vi "BackUpMove.vi"() -> ()   [LabVIEW 2017]
uses:
  <vilib>/myRIO/Instrument Drivers/Onboard IO/DIO/typedefs/DIO Reference.ctl
  <vilib>/myRIO/Common/Instrument Driver Framework/Utilities/typedefs/myRIO Generic Hardware Reference.ctl
  <vilib>/myRIO/Common/Instrument Driver Framework/Utilities/typedefs/Hardware Version Enum.ctl
  <vilib>/myRIO/Common/Instrument Driver Framework/Utilities/typedefs/myRIO v1.0 Reference.ctl
  <vilib>/myRIO/Common/Instrument Driver Framework/Utilities/typedefs/Generic FPGA Reference.ctl
  <vilib>/myRIO/Common/Instrument Driver Framework/myRIO v1.0/DIO/typedefs/DIO Channels List.ctl
  <vilib>/myRIO/Common/Instrument Driver Framework/myRIO v1.0/DIO/typedefs/DIO Channels Enum.ctl
  <vilib>/userdefined/High Color/nirio_resource_hc.ctl
  <vilib>/userdefined/High Color/IMAQdx.ctl
  <vilib>/myRIO/Common/Instrument Driver Framework/Utilities/vis/Is FPGA Ref Available.vi
  <vilib>/myRIO/Common/Instrument Driver Framework/myRIO v1.0/DIO/vis/myRIO v1.1 Open DIO.vi
  <vilib>/myRIO/Instrument Drivers/Onboard IO/DIO/vis/Write.vi
  <vilib>/myRIO/Instrument Drivers/Onboard IO/DIO/vis/Read.vi
  <vilib>/myRIO/Common/Instrument Driver Framework/Utilities/vis/Validate Channels.vi
  <vilib>/myRIO/Common/Instrument Driver Framework/myRIO v1.0/DIO/vis/myRIO v1.0 Reserve DIO.vi
  <vilib>/myRIO/Common/Instrument Driver Framework/myRIO v1.0/Resource Manager/vis/myRIO v1.0 Reserve Channel List.vi
  <vilib>/myRIO/Common/Instrument Driver Framework/myRIO v1.0/DIO/vis/myRIO v1.0 Build MUX Configuration DIO.vi
  <vilib>/myRIO/Common/Instrument Driver Framework/myRIO v1.0/Resource Manager/vis/myRIO v1.0 Reserve Channel.vi
  <vilib>/myRIO/Common/Instrument Driver Framework/myRIO v1.0/Resource Manager/vis/myRIO v1.0 Unreserve Channel.vi
  <vilib>/myRIO/Common/Instrument Driver Framework/myRIO v1.0/Resource Manager/vis/myRIO v1.0 Create Configuration List.vi
  <vilib>/myRIO/Common/Instrument Driver Framework/myRIO v1.0/Resource Manager/vis/myRIO v1.0 Build Mutex Name.vi
  <vilib>/Utility/VariantDataType/GetNumericInfo.vi
  <vilib>/Utility/error.llb/Error Cluster From Error Code.vi
  <vilib>/myRIO/Common/Instrument Driver Framework/myRIO v1.0/myRIO v1.1 Open.vi
  <vilib>/myRIO/Common/Instrument Driver Framework/Utilities/vis/IO Manager.vi
  <vilib>/myRIO/Common/Instrument Driver Framework/Utilities/vis/Configuration Manager.vi
  <vilib>/myRIO/Common/Instrument Driver Framework/myRIO v1.0/Resource Manager/vis/myRIO v1.0 Configure IO.vi
  <vilib>/myRIO/Common/Instrument Driver Framework/myRIO v1.0/myRIO v1.0 Close.vi
  <vilib>/myRIO/Common/Instrument Driver Framework/myRIO v1.0/DIO/vis/myRIO v1.0 Write DIO.vi
  <vilib>/myRIO/Common/Instrument Driver Framework/myRIO v1.0/DIO/vis/myRIO v1.0 Read DIO.vi
  Global 5.vi
  <vilib>/myRIO/Express VI/Onboard Devices/LED/LED Express VI.xnode
  <vilib>/myRIO/Instrument Drivers/Onboard IO/DIO/vis/myRIO DIO Open.xnode
  <vilib>/myRIO/Express VI/Onboard Devices/Button/Button Express VI.xnode
  <vilib>/vision/NI_Vision_Development_Module.lvlib
  <vilib>/vision/driver/NI_Vision_Acquisition_Software.lvlib
  <vilib>/myRIO/Instrument Drivers/Onboard IO/DIO/DIO.lvlib
panel:
  out "x-y":dbl
  out "Count":T1(plugin-control)
  out "Extract":T1(plugin-control)
  out "Particle":T1(plugin-control)
  out "Threshold":T1(plugin-control)
  in  "Settings":T2={"Objects"=0, "Threshold"=128, "Reject Border"=FALSE, "Fill Holes"=FALSE, "Min Object Size"=FALSE, "Min Size"=3, "Max Object Size"=FALSE, "Max Size"=100, "Show Search Area"=FALSE, "Show Center"=TRUE, "Show Bounding Box"=TRUE} {"Objects" items=["Bright Objects", "Dark Objects"]; "Threshold" min=1 max=999999999 step=1; "Max Size" min=1 max=999999999 step=1; "Min Size" min=1 max=999999999 step=1}
  in  "Number of Objects":i32
  out "Number of Objects 2":i32
  out "ROI":T3
  out "Count Encode":dbl
  out "Status":string
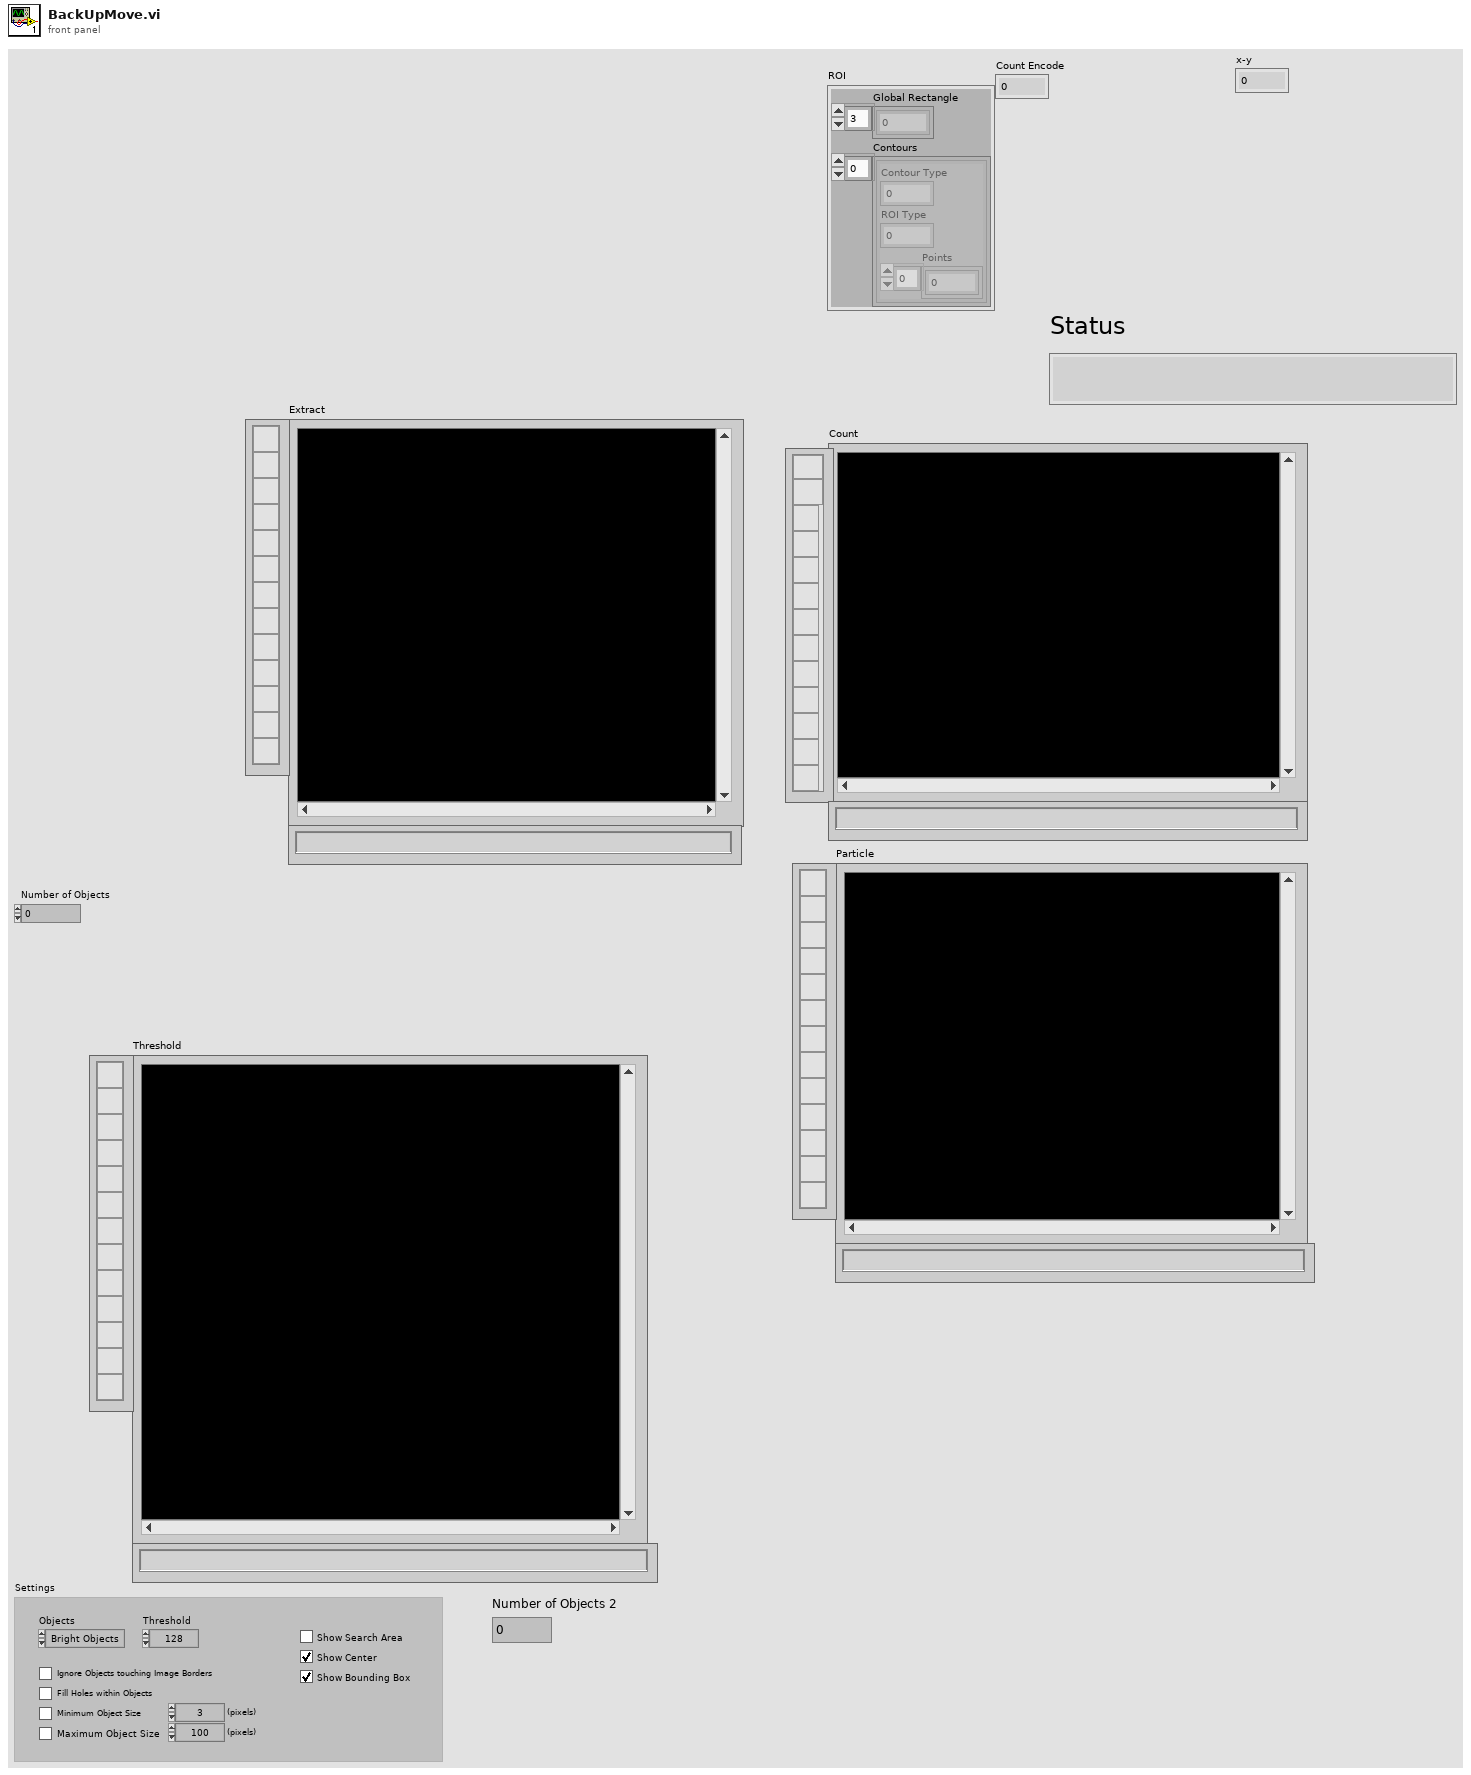
[diagram p1: front panel]
types:
  T1 = typedef "IMAQ Image.ctl" = refnum<image>
  T2 = cluster{"Objects":u16, "Threshold":i32, "Reject Border":bool, "Fill Holes":bool, "Min Object Size":bool, "Min Size":i32, "Max Object Size":bool, "Max Size":i32, "Show Search Area":bool, "Show Center":bool, "Show Bounding Box":bool}
  T3 = cluster{"Global Rectangle":i32[], "Contours":cluster{"Contour Type":u32, "ROI Type":u32, "Points":i32[]}[]}
  T4 = typedef "DIO.lvlib/DIO Reference.ctl" = cluster{"myRIO Reference":T5, "DIO Channels List":T9}
  T5 = typedef "myRIO Generic Hardware Reference.ctl" = cluster{"myRIO Model":T6, "myRIO Hardware Reference":T7}
  T6 = typedef "Hardware Version Enum.ctl" = enum16{"Unknown", "myRIO-1900", "myRIO-1950", "roboRIO", "NI ELVIS RIO CM"}
  T7 = typedef "myRIO v1.0 Reference.ctl" = cluster{"Generic FPGA Reference":T8, "Allow multiple opens":bool}
  T8 = typedef "Generic FPGA Reference.ctl" = refnum<k20>
  T9 = typedef "DIO Channels List.ctl" = T10[]
  T10 = typedef "DIO Channels Enum.ctl" = enum16{"Not Connected", "C/DIO0", "C/DIO1", "C/DIO2", "C/DIO3", "C/DIO4", "C/DIO5", "C/DIO6", "C/DIO7", "A/DIO0", "A/DIO1", "A/DIO2", "A/DIO3", "A/DIO4", "A/DIO5", "A/DIO6", "A/DIO7", "A/DIO8", "A/DIO9", "A/DIO10", "A/DIO11", "A/DIO12", "A/DIO13", "A/DIO14", "A/DIO15", "B/DIO0", "B/DIO1", "B/DIO2", "B/DIO3", "B/DIO4", "B/DIO5", "B/DIO6", "B/DIO7", "B/DIO8", "B/DIO9", "B/DIO10", "B/DIO11", "B/DIO12", "B/DIO13", "B/DIO14", "B/DIO15", "LED0", "LED1", "LED2", "LED3", "Button0", "DIO/DIO0", "DIO/DIO1", "DIO/DIO2", "DIO/DIO3", "DIO/DIO4", "DIO/DIO5", "DIO/DIO6", "DIO/DIO7", "DIO/DIO8", "DIO/DIO9", "SPI/CS0", "SPI/CS1", "SPI/CS2", "SPI/CS3", "LED RADIO (Green)", "LED RADIO (Red)", "LED COMM (Green)", "LED COMM (Red)", "LED MODE (Green)", "LED MODE (Red)"}
  T11 = typedef "nirio_resource_hc.ctl" = tag
  T12 = typedef "IMAQdx.ctl" = refnum<k21>
diagram:
  n1 = flat-sequence {
    tunnel: [w75] -> w1
    tunnel: [w156] -> w74
    tunnel: [w155] -> w73
    tunnel: [w152] -> w72
    tunnel: w1 -> [w150]
    tunnel: [w202] -> w71
    tunnel: [w201] -> w70
    tunnel: w74 -> [w202]
    tunnel: w73 -> [w201]
    tunnel: w72 -> [w200]
    tunnel: [w199] -> w69
    tunnel: w71 -> [w211]
    tunnel: w70 -> [w210]
    tunnel: [w211] -> w68
    tunnel: [w210] -> w67
    tunnel: w69 -> [w209]
    tunnel: [w208] -> w66
    tunnel: [w221] -> w65
    tunnel: [w220] -> w64
    tunnel: w68 -> [w221]
    tunnel: w67 -> [w220]
    tunnel: w66 -> [w217]
    tunnel: [w215] -> w63
    tunnel: w65 -> [w230]
    tunnel: w64 -> [w229]
    tunnel: [w230] -> w61
    tunnel: [w229] -> w62
    tunnel: w63 -> [w228]
    tunnel: [w227] -> w60
    tunnel: w62 -> [w237]
    tunnel: [w237] -> w59
    tunnel: w61 -> [w236]
    tunnel: [w236] -> w58
    tunnel: [w234] -> w57
    tunnel: w60 -> [w234]
    tunnel: w59 -> [w244]
    tunnel: w58 -> [w243]
    tunnel: [w244] -> w56
    tunnel: [w243] -> w55
    tunnel: w57 -> [w240]
    tunnel: [w238] -> w54
    tunnel: w56 -> [w252]
    tunnel: w55 -> [w253]
    tunnel: [w253] -> w53
    tunnel: [w252] -> w52
    tunnel: w54 -> [w251]
    tunnel: [w250] -> w51
    tunnel: [w260] -> w50
    tunnel: w53 -> [w260]
    tunnel: [w259] -> w49
    tunnel: w52 -> [w259]
    tunnel: [w257] -> w48
    tunnel: w51 -> [w257]
    tunnel: [w264] -> w47
    tunnel: [w266] -> w46
    tunnel: w50 -> [w266]
    tunnel: w49 -> [w264]
    tunnel: w48 -> [w263]
    tunnel: [w262] -> w45
    tunnel: w47 -> [w311]
    tunnel: w46 -> [w312]
    tunnel: [w312] -> w44
    tunnel: [w311] -> w43
    tunnel: w45 -> [w310]
    tunnel: [w309] -> w42
    tunnel: [w355] -> w41
    tunnel: [w356] -> w40
    tunnel: w44 -> [w356]
    tunnel: w43 -> [w355]
    tunnel: w42 -> [w353]
    tunnel: [w351] -> w39
    tunnel: w41 -> [w364]
    tunnel: w40 -> [w365]
    tunnel: w39 -> [w367]
    tunnel: [w366] -> w38
    tunnel: [w365] -> w37
    tunnel: [w364] -> w36
    tunnel: [w372] -> w35
    tunnel: [w373] -> w34
    tunnel: w38 -> [w376]
    tunnel: w37 -> [w375]
    tunnel: w36 -> [w374]
    tunnel: [w371] -> w33
    tunnel: [w435] -> w32
    tunnel: [w436] -> w31
    tunnel: w35 -> [w435]
    tunnel: w34 -> [w433]
    tunnel: [w431] -> w30
    tunnel: w33 -> [w436]
    tunnel: w32 -> [w446]
    tunnel: w31 -> [w445]
    tunnel: [w445] -> w29
    tunnel: [w446] -> w28
    tunnel: [w445] -> w27
    tunnel: w30 -> [w444]
    tunnel: [w443] -> w26
    tunnel: w29 -> [_]
    tunnel: w28 -> [w452]
    tunnel: [w452] -> w25
    tunnel: [w451] -> w24
    tunnel: w27 -> [w451]
    tunnel: w26 -> [w450]
    tunnel: [w450] -> w23
    tunnel: w25 -> [w458]
    tunnel: w24 -> [w459]
    tunnel: [w459] -> w22
    tunnel: [w458] -> w21
    tunnel: w23 -> [w456]
    tunnel: [w454] -> w20
    tunnel: w22 -> [w467]
    tunnel: w21 -> [w466]
    tunnel: w20 -> [w469]
    tunnel: [w468] -> w4
    tunnel: [w467] -> w3
    tunnel: [w466] -> w2
    tunnel: [w478] -> w19
    tunnel: [w473] -> w18
    tunnel: [w474] -> w17
    tunnel: w4 -> [w475]
    tunnel: w3 -> [w474]
    tunnel: w2 -> [w473]
    tunnel: w19 -> [w490]
    tunnel: [w489] -> w16
    tunnel: w18 -> [w488]
    tunnel: [w488] -> w15
    tunnel: w17 -> [w487]
    tunnel: [w487] -> w14
    tunnel: w16 -> [w495]
    tunnel: w15 -> [w497]
    tunnel: w14 -> [w496]
    tunnel: [w497] -> w13
    tunnel: [w496] -> w12
    tunnel: [w495] -> w11
    tunnel: w13 -> [w508]
    tunnel: [w508] -> w10
    tunnel: w12 -> [w507]
    tunnel: [w507] -> w9
    tunnel: w11 -> [w506]
    tunnel: [w505] -> w8
    tunnel: w10 -> [w515]
    tunnel: w9 -> [w514]
    tunnel: w8 -> [w517]
    tunnel: [w515] -> w7
    tunnel: [w514] -> w6
    tunnel: [w513] -> w5
    tunnel: w7 -> [w563]
    tunnel: w6 -> [w562]
    tunnel: w5 -> [w561]
    frame #0 {
      n2 = while {
        tunnel: [w76] -> w75
        stop <- w78 stop-if-true
        n3 = xnode "Start"("LED0"=TRUE) -> ("error out"=w77:errorcluster)  [unwired: 1 in]
        n4 = xnode "Button"("error in (no error)"=w77) -> ("Value"=w78:bool, "error out"=w76:errorcluster)
      }
    }
    frame #1 {
      w156 = tag "B/I2C" ("myRIO MXP Port A/B")
      w155 = u8 1 ("Controller ID#  (I2C Address)")
      # "enable"
      n5 = Wait (ms)(milliseconds to wait=u32 1000) -> ()  [unwired: 1 out]
      n6 = local write "Status"("Starting" ("Status")) -> ()
      n7 = xnode "Start 2"("LED0"=FALSE) -> ()  [unwired: 1 in, 1 out]
      n8 = call <vilib>:"TETRIX_Enable_DC_Controller_myRIO.vi"("myRIO MXP Port A/B"=w156, "Controller ID#  (I2C Address)"=w155, "Error/Flow In"=w150) -> ("Error/Flow Out"=w154:errorcluster)  [unwired: 4 in]
      n9 = call <vilib>:"TETRIX_Motor_Invert_myRIO.vi"("myRIO MXP Port A/B"=w156, "Invert State"=TRUE, "Select Channel"="Motor 1", "Controller ID#  (I2C Address)"=w155) -> ()  [unwired: 3 in, 1 out]
      n10 = call <vilib>:"TETRIX_Reset_Encoders_myRIO.vi"("myRIO MXP Port A/B"=w156, "Select Encoder"="Encoders 1 and 2", "Controller ID#  (I2C Address)"=w155, "Error/Flow In"=w154) -> ("Error/Flow Out"=w153:errorcluster)  [unwired: 3 in]
      n11 = call <vilib>:"TETRIX_Stop_Motors_myRIO.vi"("myRIO MXP Port A/B"=w156, "Stop Mode"="Brake", "Select Channel"="Both Motors", "Controller ID#  (I2C Address)"=w155, "Error/Flow In"=w153) -> ("Error/Flow Out"=w152:errorcluster)  [unwired: 2 in]
    }
    frame #2 {
      w204 = 700 ("Motor 2 Encoder Target")
      w206 = i16 200 ("Motor 1 Contant Speed (Degrees per Second)")
      # "fate 1 start position"
      n12 = Wait (ms)(milliseconds to wait=u32 5500) -> ()  [unwired: 1 out]
      n13 = call <vilib>:"TETRIX_Set_Motor_Target(s)_myRIO.vi"("Motor 2 Encoder Target"=w204, "Motor 1 Encoder Target"=w204, "myRIO MXP Port A/B"=w202, "Controller ID#  (I2C Address)"=w201, "Motor 2 Constant Speed (Degrees per Second)"=w206, "Motor 1 Contant Speed (Degrees per Second)"=w206, "Encoder Units"="Degrees", "Error/Flow In"=w200) -> ("Error/Flow Out"=w199:errorcluster)  [unwired: 1 in]
      "Status" <- "Phase 1" ("Status")
    }
    frame #3 {
      n14 = Wait (ms)(milliseconds to wait=u32 500) -> ()  [unwired: 1 out]
      n15 = call <vilib>:"TETRIX_Stop_Motors_myRIO.vi"("myRIO MXP Port A/B"=w211, "Stop Mode"="Brake", "Select Channel"="Both Motors", "Controller ID#  (I2C Address)"=w210, "Error/Flow In"=w209) -> ("Error/Flow Out"=w208:errorcluster)  [unwired: 2 in]
    }
    frame #4 {
      w226 = i16 100 ("Motor 1 Contant Speed (Degrees per Second)")
      # "fate 2 catch ball"
      n16 = Wait (ms)(milliseconds to wait=u32 3000) -> ()  [unwired: 1 out]
      n17 = local write "Status"("Turning" ("Status")) -> ()
      n18 = call <vilib>:"TETRIX_Reset_Encoders_myRIO.vi"("myRIO MXP Port A/B"=w221, "Select Encoder"="Encoders 1 and 2", "Controller ID#  (I2C Address)"=w220, "Error/Flow In"=w217) -> ("Error/Flow Out"=w216:errorcluster)  [unwired: 3 in]
      n19 = call <vilib>:"TETRIX_Set_Motor_Target(s)_myRIO.vi"("Motor 2 Encoder Target"=300 ("Motor 1 Encoder Target"), "Motor 1 Encoder Target"=-290, "myRIO MXP Port A/B"=w221, "Controller ID#  (I2C Address)"=w220, "Motor 2 Constant Speed (Degrees per Second)"=w226, "Motor 1 Contant Speed (Degrees per Second)"=w226, "Encoder Units"="Degrees", "Error/Flow In"=w216) -> ("Error/Flow Out"=w215:errorcluster)  [unwired: 1 in]
    }
    frame #5 {
      n20 = Wait (ms)(milliseconds to wait=u32 500) -> ()  [unwired: 1 out]
      n21 = call <vilib>:"TETRIX_Stop_Motors_myRIO.vi"("myRIO MXP Port A/B"=w230, "Stop Mode"="Brake", "Select Channel"="Both Motors", "Controller ID#  (I2C Address)"=w229, "Error/Flow In"=w228) -> ("Error/Flow Out"=w227:errorcluster)  [unwired: 2 in]
    }
    frame #6 {
      n22 = local write "Status"("Move Gripper" ("Status")) -> ()
      n23 = call "ServoPickup.vi"() -> ()  [unwired: 12 in]
    }
    frame #7 {
      w246 = i16 100 ("Motor 1 Contant Speed (Degrees per Second)")
      n24 = Wait (ms)(milliseconds to wait=u32 5000) -> ()  [unwired: 1 out]
      n25 = local write "Status"("Moving to catch" ("Status")) -> ()
      n26 = call <vilib>:"TETRIX_Reset_Encoders_myRIO.vi"("myRIO MXP Port A/B"=w243, "Select Encoder"="Encoders 1 and 2", "Controller ID#  (I2C Address)"=w244, "Error/Flow In"=w240) -> ("Error/Flow Out"=w239:errorcluster)  [unwired: 3 in]
      n27 = call <vilib>:"TETRIX_Set_Motor_Target(s)_myRIO.vi"("Motor 2 Encoder Target"=420 ("Motor 1 Encoder Target"), "Motor 1 Encoder Target"=420, "myRIO MXP Port A/B"=w243, "Controller ID#  (I2C Address)"=w244, "Motor 2 Constant Speed (Degrees per Second)"=w246, "Motor 1 Contant Speed (Degrees per Second)"=w246, "Encoder Units"="Degrees", "Error/Flow In"=w239) -> ("Error/Flow Out"=w238:errorcluster)  [unwired: 1 in]
    }
    frame #8 {
      n28 = Wait (ms)(milliseconds to wait=u32 500) -> ()  [unwired: 1 out]
      n29 = call <vilib>:"TETRIX_Stop_Motors_myRIO.vi"("myRIO MXP Port A/B"=w253, "Stop Mode"="Brake", "Select Channel"="Both Motors", "Controller ID#  (I2C Address)"=w252, "Error/Flow In"=w251) -> ("Error/Flow Out"=w250:errorcluster)  [unwired: 2 in]
    }
    frame #9 {
      n30 = local write "Status"("Catching" ("Status")) -> ()
      n31 = call "PickBall.vi"() -> ()  [unwired: 12 in]
    }
    frame #10 {
      w269 = i16 100 ("Motor 1 Contant Speed (Degrees per Second)")
      n32 = Wait (ms)(milliseconds to wait=u32 4200) -> ()  [unwired: 1 out]
      n33 = xnode "LED"("LED1"=TRUE) -> ()  [unwired: 1 in, 1 out]
      n34 = call <vilib>:"TETRIX_Set_Motor_Target(s)_myRIO.vi"("Motor 2 Encoder Target"=300 ("Motor 1 Encoder Target"), "Motor 1 Encoder Target"=300, "myRIO MXP Port A/B"=w266, "Controller ID#  (I2C Address)"=w264, "Motor 2 Constant Speed (Degrees per Second)"=w269, "Motor 1 Contant Speed (Degrees per Second)"=w269, "Encoder Units"="Degrees", "Error/Flow In"=w263) -> ("Error/Flow Out"=w262:errorcluster)  [unwired: 1 in]
      n35 = local write "Status"("Moving to Bowling" ("Status")) -> ()
      n36 = call <vilib>:"TETRIX_Reset_Encoders_myRIO.vi"("myRIO MXP Port A/B"=w266, "Select Encoder"="Encoders 1 and 2", "Controller ID#  (I2C Address)"=w264) -> ()  [unwired: 4 in, 1 out]
    }
    frame #11 {
      # "end fate2"
      n37 = Wait (ms)(milliseconds to wait=u32 500) -> ()  [unwired: 1 out]
      n38 = xnode "LED 2"("LED1"=FALSE) -> ()  [unwired: 1 in, 1 out]
      n39 = call <vilib>:"TETRIX_Stop_Motors_myRIO.vi"("myRIO MXP Port A/B"=w312, "Stop Mode"="Brake", "Select Channel"="Both Motors", "Controller ID#  (I2C Address)"=w311, "Error/Flow In"=w310) -> ("Error/Flow Out"=w309:errorcluster)  [unwired: 2 in]
    }
    frame #12 {
      w360 = i16 100 ("Motor 2 Constant Speed (Degrees per Second)")
      # "fate 3  go to shoot ball position"
      n40 = Wait (ms)(milliseconds to wait=u32 3000) -> ()  [unwired: 1 out]
      n41 = local write "Status"("Phase 3 Turning" ("Status")) -> ()
      n42 = call <vilib>:"TETRIX_Reset_Encoders_myRIO.vi"("myRIO MXP Port A/B"=w356, "Select Encoder"="Encoders 1 and 2", "Controller ID#  (I2C Address)"=w355, "Error/Flow In"=w353) -> ("Error/Flow Out"=w352:errorcluster)  [unwired: 3 in]
      n43 = call <vilib>:"TETRIX_Set_Motor_Target(s)_myRIO.vi"("Motor 2 Encoder Target"=300, "Motor 1 Encoder Target"=-315, "myRIO MXP Port A/B"=w356, "Controller ID#  (I2C Address)"=w355, "Motor 2 Constant Speed (Degrees per Second)"=w360, "Motor 1 Contant Speed (Degrees per Second)"=w360, "Encoder Units"="Degrees", "Error/Flow In"=w352) -> ("Error/Flow Out"=w351:errorcluster)  [unwired: 1 in]
    }
    frame #13 {
      n44 = Wait (ms)(milliseconds to wait=u32 500) -> ()  [unwired: 1 out]
      n45 = global write "Global 5.vi" "Count Encode"(50.0 ("Count Encode")) -> ()
      n46 = call <vilib>:"TETRIX_Stop_Motors_myRIO.vi"("myRIO MXP Port A/B"=w365, "Stop Mode"="Brake", "Select Channel"="Both Motors", "Controller ID#  (I2C Address)"=w364, "Error/Flow In"=w367) -> ("Error/Flow Out"=w366:errorcluster)  [unwired: 2 in]
    }
    frame #14 {
      (unwired) "im0" ("Image Name")
      n47 = call "IMAQ Create"("Image Name"="im0") -> ("New Image"=w380:T1)  [unwired: 4 in, 1 out]
      n48 = call "IMAQ Create"("Image Name"="im1") -> ("New Image"=w378:T1)  [unwired: 4 in, 1 out]
      n49 = while {
        tunnel: w380 -> [w408]
        tunnel: w378 -> [w405]
        tunnel: w374 -> [w401]
        tunnel: w376 -> [w389]
        tunnel: w375 -> [w384]
        tunnel: [w387] -> w373
        tunnel: [w385] -> w372
        tunnel: [w382] -> w371
        stop <- w399 stop-if-true
        w409 = u16 1 items=["RGB", "HSL", "HSV", "HSI"] ("Color Mode")
        n50 = flat-sequence {
          tunnel: w401 -> [w413]
          tunnel: w389 -> [w418]
          tunnel: [w416] -> w388
          tunnel: [w413] -> w386
          tunnel: w384 -> [w412]
          tunnel: [w412] -> w383
          tunnel: w388 -> [w427]
          tunnel: [w426] -> w387
          tunnel: w386 -> [w425]
          tunnel: [w425] -> w385
          tunnel: w383 -> [w424]
          tunnel: [w424] -> w382
          frame #0 {
            w415 = 50 ("Motor 1 Encoder Target")
            w421 = i16 100 ("Motor 1 Contant Speed (Degrees per Second)")
            n51 = global read "Global 5.vi" "Count Encode"() -> (w419:dbl)
            n52 = Wait (ms)(milliseconds to wait=u32 500 ("millisecond timer value")) -> ()  [unwired: 1 out]
            n53 = Add(x=50.0, y=w419) -> (x+y=w411:dbl)
            "Count Encode" <- w411
            n54 = call <vilib>:"TETRIX_Reset_Encoders_myRIO.vi"("myRIO MXP Port A/B"=w412, "Select Encoder"="Encoders 1 and 2", "Controller ID#  (I2C Address)"=w413, "Error/Flow In"=w418) -> ("Error/Flow Out"=w417:errorcluster)  [unwired: 3 in]
            n55 = call <vilib>:"TETRIX_Set_Motor_Target(s)_myRIO.vi"("Motor 2 Encoder Target"=w415, "Motor 1 Encoder Target"=w415, "myRIO MXP Port A/B"=w412, "Controller ID#  (I2C Address)"=w413, "Motor 2 Constant Speed (Degrees per Second)"=w421, "Motor 1 Contant Speed (Degrees per Second)"=w421, "Encoder Units"="Degrees", "Error/Flow In"=w417) -> ("Error/Flow Out"=w416:errorcluster)  [unwired: 1 in]
            n56 = global write "Global 5.vi" "Count Encode"(w411) -> ()
          }
          frame #1 {
            n57 = Wait (ms)(milliseconds to wait=u32 500 ("millisecond timer value")) -> ()  [unwired: 1 out]
            n58 = call <vilib>:"TETRIX_Stop_Motors_myRIO.vi"("myRIO MXP Port A/B"=w424, "Stop Mode"="Brake", "Select Channel"="Both Motors", "Controller ID#  (I2C Address)"=w425, "Error/Flow In"=w427) -> ("Error/Flow Out"=w426:errorcluster)  [unwired: 2 in]
          }
        }
        n59 = property on="Count" class="ImageControl"() -> ("ROI"=→"ROI":T3)  [unwired: 2 in, 2 out]
        n60 = call <vilib>:"IMAQdx Snap2.vi"("Image In"=w408, "Session In"=T12 "cam0") -> ("Image Out"=w410:T1)  [unwired: 7 in, 2 out]
        n61 = call "IMAQ ExtractColorPlanes"("Blue or Luma or Val or Inten Plane"=w405, "Color Mode"=w409, "Image Src"=w410) -> ("Blue or Luma or Val or Inten Plane out"=w406:T1)  [unwired: 5 in, 3 out]
        n62 = call "IMAQ Rotate"("Angle (degrees)"=sgl -2.3, "Image Src"=w406) -> ("Image Dst Out"=w395:T1)  [unwired: 8 in, 1 out]
        "Count" <- w395
        n63 = call "IMAQ Extract 2"("Optional Rectangle"=i32[] [327, 228, 351, 263], "Image Src"=w395) -> ("Image Dst Out"=w404:T1)  [unwired: 8 in, 1 out]
        "Extract" <- w404
        "Particle" <- w404
        n64 = global read "Global 5.vi" "Count Encode"() -> (w398:dbl)
        n65 = call "IMAQ Count Objects 2"("Settings"="Settings", "Image"=w404) -> ("Number of Objects"=w392:i32, "Image Out"=→"Threshold":T1)  [unwired: 5 in, 3 out]
        "Number of Objects 2" <- w392
        n66 = Greater?(x=w392, y=2) -> (0:w393:bool)
        n67 = Greater Or Equal?(x=w398, y=1200.0) -> (x >= y?=w396:bool)
        n68 = Or(x=w393, y=w396) -> (x .or. y?=w399:bool)
      }
      n69 = local write "Status"("IMAQ Start" ("Status")) -> ()
    }
    frame #15 {
      w441 = i16 100 ("Motor 1 Contant Speed (Degrees per Second)")
      n70 = Wait (ms)(milliseconds to wait=u32 3000) -> ()  [unwired: 1 out]
      n71 = local write "Status"("Turning to shoot" ("Status")) -> ()
      n72 = call <vilib>:"TETRIX_Reset_Encoders_myRIO.vi"("myRIO MXP Port A/B"=w436, "Select Encoder"="Encoders 1 and 2", "Controller ID#  (I2C Address)"=w435, "Error/Flow In"=w433) -> ("Error/Flow Out"=w432:errorcluster)  [unwired: 3 in]
      n73 = call <vilib>:"TETRIX_Set_Motor_Target(s)_myRIO.vi"("Motor 2 Encoder Target"=-285, "Motor 1 Encoder Target"=290, "myRIO MXP Port A/B"=w436, "Controller ID#  (I2C Address)"=w435, "Motor 2 Constant Speed (Degrees per Second)"=w441, "Motor 1 Contant Speed (Degrees per Second)"=w441, "Encoder Units"="Degrees", "Error/Flow In"=w432) -> ("Error/Flow Out"=w431:errorcluster)  [unwired: 1 in]
    }
    frame #16 {
      n74 = Wait (ms)(milliseconds to wait=u32 500) -> ()  [unwired: 1 out]
      n75 = call <vilib>:"TETRIX_Stop_Motors_myRIO.vi"("myRIO MXP Port A/B"=w445, "Stop Mode"="Brake", "Select Channel"="Both Motors", "Controller ID#  (I2C Address)"=w446, "Error/Flow In"=w444) -> ("Error/Flow Out"=w443:errorcluster)  [unwired: 2 in]
    }
    frame #17 {
      # "fate 4 shoot ball"
      n76 = local write "Status"(" Shooting" ("Status")) -> ()
      n77 = call "Shoot.vi"() -> ()  [unwired: 12 in]
    }
    frame #18 {
      w464 = i16 100 ("Motor 1 Contant Speed (Degrees per Second)")
      n78 = Wait (ms)(milliseconds to wait=u32 3000) -> ()  [unwired: 1 out]
      n79 = local write "Status"("Turning to Check" ("Status")) -> ()
      n80 = call <vilib>:"TETRIX_Reset_Encoders_myRIO.vi"("myRIO MXP Port A/B"=w459, "Select Encoder"="Encoders 1 and 2", "Controller ID#  (I2C Address)"=w458, "Error/Flow In"=w456) -> ("Error/Flow Out"=w455:errorcluster)  [unwired: 3 in]
      n81 = call <vilib>:"TETRIX_Set_Motor_Target(s)_myRIO.vi"("Motor 2 Encoder Target"=300, "Motor 1 Encoder Target"=-285, "myRIO MXP Port A/B"=w459, "Controller ID#  (I2C Address)"=w458, "Motor 2 Constant Speed (Degrees per Second)"=w464, "Motor 1 Contant Speed (Degrees per Second)"=w464, "Encoder Units"="Degrees", "Error/Flow In"=w455) -> ("Error/Flow Out"=w454:errorcluster)  [unwired: 1 in]
    }
    frame #19 {
      n82 = Wait (ms)(milliseconds to wait=u32 500) -> ()  [unwired: 1 out]
      n83 = call <vilib>:"TETRIX_Stop_Motors_myRIO.vi"("myRIO MXP Port A/B"=w467, "Stop Mode"="Brake", "Select Channel"="Both Motors", "Controller ID#  (I2C Address)"=w466, "Error/Flow In"=w469) -> ("Error/Flow Out"=w468:errorcluster)  [unwired: 2 in]
    }
    frame #20 {
      w484 = i16 200 ("Motor 1 Contant Speed (Degrees per Second)")
      n84 = call <vilib>:"TETRIX_Reset_Encoders_myRIO.vi"("myRIO MXP Port A/B"=w474, "Select Encoder"="Encoders 1 and 2", "Controller ID#  (I2C Address)"=w473, "Error/Flow In"=w475) -> ("Error/Flow Out"=w485:errorcluster)  [unwired: 3 in]
      n85 = Wait (ms)(milliseconds to wait=u32 5000) -> ()  [unwired: 1 out]
      n86 = global read "Global 5.vi" "Count Encode"() -> (w481:dbl)
      n87 = local write "Status"("Encode to Home " ("Status")) -> ()
      n88 = Subtract(x=870.0, y=w481) -> (x-y=w479:dbl)
      "x-y" <- w479
      n89 = call <vilib>:"TETRIX_Set_Motor_Target(s)_myRIO.vi"("Motor 2 Encoder Target"=w479, "Motor 1 Encoder Target"=w479, "myRIO MXP Port A/B"=w474, "Controller ID#  (I2C Address)"=w473, "Motor 2 Constant Speed (Degrees per Second)"=w484, "Motor 1 Contant Speed (Degrees per Second)"=w484, "Encoder Units"="Degrees", "Error/Flow In"=w485) -> ("Error/Flow Out"=w478:errorcluster)  [unwired: 1 in]
    }
    frame #21 {
      n90 = call <vilib>:"TETRIX_Stop_Motors_myRIO.vi"("myRIO MXP Port A/B"=w487, "Stop Mode"="Brake", "Select Channel"="Both Motors", "Controller ID#  (I2C Address)"=w488, "Error/Flow In"=w490) -> ("Error/Flow Out"=w489:errorcluster)  [unwired: 2 in]
      n91 = Wait (ms)(milliseconds to wait=u32 500) -> ()  [unwired: 1 out]
    }
    frame #22 {
      w502 = i16 100 ("Motor 1 Contant Speed (Degrees per Second)")
      n92 = call <vilib>:"TETRIX_Reset_Encoders_myRIO.vi"("myRIO MXP Port A/B"=w496, "Select Encoder"="Encoders 1 and 2", "Controller ID#  (I2C Address)"=w497, "Error/Flow In"=w495) -> ("Error/Flow Out"=w499:errorcluster)  [unwired: 3 in]
      n93 = local write "Status"("Turning" ("Status")) -> ()
      n94 = Wait (ms)(milliseconds to wait=u32 4500) -> ()  [unwired: 1 out]
      n95 = call <vilib>:"TETRIX_Set_Motor_Target(s)_myRIO.vi"("Motor 2 Encoder Target"=290, "Motor 1 Encoder Target"=-295, "myRIO MXP Port A/B"=w496, "Controller ID#  (I2C Address)"=w497, "Motor 2 Constant Speed (Degrees per Second)"=w502, "Motor 1 Contant Speed (Degrees per Second)"=w502, "Encoder Units"="Degrees", "Error/Flow In"=w499) -> ()  [unwired: 1 in, 1 out]
    }
    frame #23 {
      n96 = call <vilib>:"TETRIX_Stop_Motors_myRIO.vi"("myRIO MXP Port A/B"=w507, "Stop Mode"="Brake", "Select Channel"="Both Motors", "Controller ID#  (I2C Address)"=w508, "Error/Flow In"=w506) -> ("Error/Flow Out"=w505:errorcluster)  [unwired: 2 in]
      n97 = Wait (ms)(milliseconds to wait=u32 500) -> ()  [unwired: 1 out]
    }
    frame #24 {
      w521 = i16 200 ("Motor 1 Contant Speed (Degrees per Second)")
      n98 = call <vilib>:"TETRIX_Reset_Encoders_myRIO.vi"("myRIO MXP Port A/B"=w514, "Select Encoder"="Encoders 1 and 2", "Controller ID#  (I2C Address)"=w515, "Error/Flow In"=w517) -> ("Error/Flow Out"=w516:errorcluster)  [unwired: 3 in]
      n99 = Wait (ms)(milliseconds to wait=u32 8000) -> ()  [unwired: 1 out]
      n100 = xnode "END 2"("LED3"=FALSE) -> ()  [unwired: 1 in, 1 out]
      n101 = call <vilib>:"TETRIX_Set_Motor_Target(s)_myRIO.vi"("Motor 2 Encoder Target"=900, "Motor 1 Encoder Target"=900, "myRIO MXP Port A/B"=w514, "Controller ID#  (I2C Address)"=w515, "Motor 2 Constant Speed (Degrees per Second)"=w521, "Motor 1 Contant Speed (Degrees per Second)"=w521, "Encoder Units"="Degrees", "Error/Flow In"=w516) -> ("Error/Flow Out"=w513:errorcluster)  [unwired: 1 in]
    }
    frame #25 {
      n102 = xnode "END"("LED3"=TRUE) -> ()  [unwired: 1 in, 1 out]
      n103 = local write "Status"("Welcome Home" ("Status")) -> ()
      n104 = Wait (ms)(milliseconds to wait=u32 500) -> ()  [unwired: 1 out]
      n105 = call <vilib>:"TETRIX_Stop_Motors_myRIO.vi"("myRIO MXP Port A/B"=w562, "Stop Mode"="Brake", "Select Channel"="Both Motors", "Controller ID#  (I2C Address)"=w563, "Error/Flow In"=w561) -> ()  [unwired: 2 in, 1 out]
    }
  }
